vi "Stop Core.vi"(10 "final error code":i32 caption="最终错误代码", 11 "生命游戏 in":refnum<class "生命游戏.lvclass"> caption="操作者输入") -> (3 "生命游戏 out":refnum<class "生命游戏.lvclass"> caption="操作者输出")   [LabVIEW 2015, in "生命游戏.lvlib" / "生命游戏.lvclass"]
doc: "(<B>文件名</B>: Actor Framework.lvlib:Actor.lvclass:Stop Core.vi)\n\n定义停止前操作者的动作。Use the <B>final error code</B> input to determine whether the actor shut down in response to an error.\n\nBy default, this method passes the Stop message along to all auto-stop nested actors.A descendant class may override this method to define additional behavior, such as shutting down any processes the actor initiated in its override of the Actor Core method."
uses:
  <vilib>/ActorFramework/Actor/Actor.lvclass
  <vilib>/ActorFramework/Time-Delayed Send Message/Time-Delay Override Options.ctl
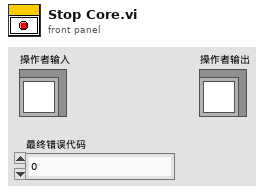
[diagram p1: front panel]
types:
  T1 = typedef "Time-Delay Override Options.ctl" = enum16{"Send next copy now", "Skip next scheduled copy", "Send next copy now and stop all further copies", "Stop all further copies"}
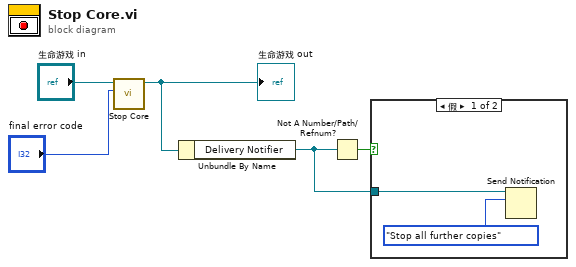
[diagram p0: block diagram]
diagram:
  n1 = call-parent "Stop Core.vi"("final error code"="final error code", "Actor in"="生命游戏 in") -> ("Actor out"=w3:refnum<class "生命游戏.lvclass">)  [unwired: 9 in]
  "生命游戏 out" <- w3
  n2 = Unbundle By Name(w3) -> ("Delivery Notifier"=w1:refnum<notifier>)
  n3 = Not A Number/Path/Refnum?(number/path/refnum=w1) -> (NaN/Path/Refnum?=w2:bool)
  n4 = case shown="假" w2 {
    tunnel: w1 -> [w7 _]
    frame False {
      n5 = Send Notification(notification=Time-Delay_Override_Options."Stop all further copies" ("通知"), notifier=w7) -> ()  [unwired: 1 in, 2 out]
    }
    frame True {
    }
  }
